vi "Temperature conversion.vi"() -> ()   [LabVIEW 2014]
panel:
  out "TEMP C":dbl
  out "TEMP F":dbl
  in  "Slide":dbl(slide) scale=0.0..100.0
  out "Thermometer (C)":dbl(slide) scale=0.0..100.0
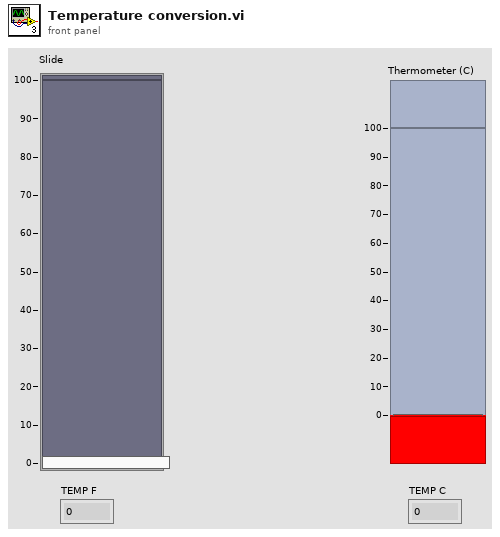
[diagram p1: front panel]
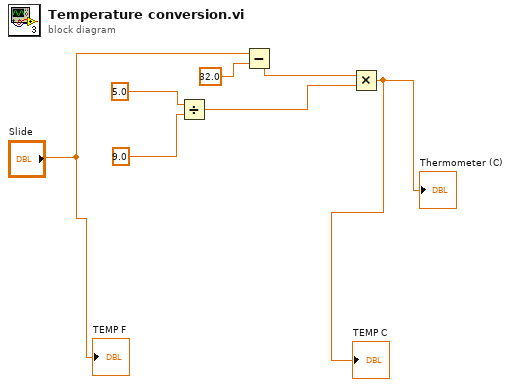
[diagram p0: block diagram]
diagram:
  n1 = Divide(x=5.0, y=9.0) -> (x/y=w5:dbl)
  n2 = Subtract(x="Slide", y=32.0) -> (x-y=w6:dbl)
  n3 = Multiply(x=w6, y=w5) -> (x*y=→"Thermometer (C)" →"TEMP C":dbl)
  "TEMP F" <- "Slide"
